vi "ISR.vi"(11 "IRQ Number":u8) -> ()   [LabVIEW 2021]
uses:
  rpmMeasGlobals.vi
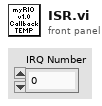
[diagram p1: front panel]
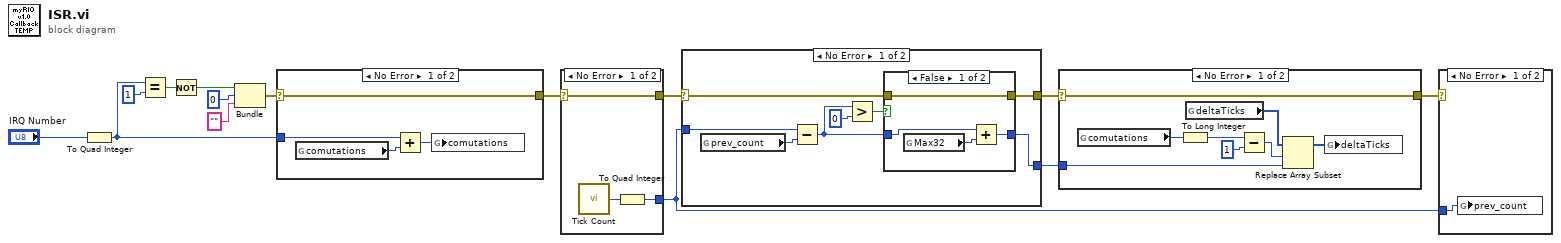
[diagram p0: block diagram]
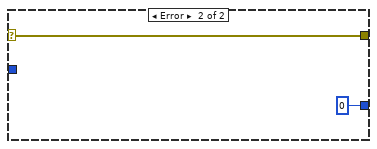
[diagram p3: hidden frame]
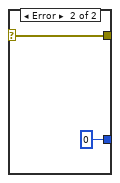
[diagram p4: hidden frame]
diagram:
  n1 = To Quad Integer(1:"IRQ Number") -> (0:w10:i64)
  n2 = Equal?(x=w10, y=i64 1) -> (x = y?=w5:bool)
  n3 = Not(x=w5) -> (.not. x?=w4:bool)
  n4 = Bundle(w4, "code"=0, "source"="") -> (w9:cluster{bool, "code":i32, "source":string})  [unwired: 1 in]
  n5 = case shown="No Error" w9 {
    selector: w9 -> [w16 w19]
    tunnel: w10 -> [w17 _]
    tunnel: [w16 w19] -> w3
    frame No Error {
      n6 = global read "rpmMeasGlobals.vi" "comutations"() -> (w15:i64)
      n7 = Add(x=w17, y=w15) -> (x+y=w18:i64)
      n8 = global write "rpmMeasGlobals.vi" "comutations"(w18) -> ()
    }
    frame Error {
    }
  }
  n9 = case shown="No Error" w3 {
    selector: w3 -> [w22 w24]
    tunnel: [w22 w24] -> w1
    tunnel: [w20 i64 0] -> w2
    frame No Error {
      n10 = call "Tick Count"() -> ("Tick Count(uSec)"=w21:u32)
      n11 = To Quad Integer(1:w21) -> (0:w20:i64)
    }
    frame Error {
    }
  }
  n12 = case shown="No Error" w1 {
    selector: w1 -> [w25 w40]
    tunnel: [w29 w40] -> w8
    tunnel: [w28 i64 0] -> w7
    tunnel: w2 -> [w26 _]
    frame No Error {
      n13 = global read "rpmMeasGlobals.vi" "prev_count"() -> (w32:i64)
      n14 = Subtract(x=w26, y=w32) -> (x-y=w30:i64)
      n15 = Greater?(x=w30, y=i64 0) -> (0:w27:bool)
      n16 = case shown="False" w27 {
        tunnel: w30 -> [w35 w38]
        tunnel: [w34 w38] -> w28
        tunnel: [w33 w37] -> w29
        tunnel: w25 -> [w33 w37]
        frame False {
          n17 = global read "rpmMeasGlobals.vi" "Max32"() -> (w36:i64)
          n18 = Add(x=w35, y=w36) -> (x+y=w34:i64)
        }
        frame True {
        }
      }
    }
    frame Error {
    }
  }
  n19 = case shown="No Error" w8 {
    selector: w8 -> [w48 w49]
    tunnel: w7 -> [w45 _]
    tunnel: [w48 w49] -> w6
    frame No Error {
      n20 = global read "rpmMeasGlobals.vi" "comutations"() -> (w44:i64)
      n21 = To Long Integer(number=w44) -> (32bit integer=w43:i32)
      n22 = global read "rpmMeasGlobals.vi" "deltaTicks"() -> (w47:i64[])
      n23 = Subtract(x=w43, y=1) -> (x-y=w41:i32)
      n24 = Replace Array Subset(array=w47, new element=w45, index=w41) -> (w46:i64[])
      n25 = global write "rpmMeasGlobals.vi" "deltaTicks"(w46) -> ()
    }
    frame Error {
    }
  }
  n26 = case shown="No Error" w6 {
    tunnel: w2 -> [w50 _]
    frame No Error {
      n27 = global write "rpmMeasGlobals.vi" "prev_count"(w50) -> ()
    }
    frame Error {
    }
  }
